vi "List-ALL-subfolders-and-files-1D.vi"(7 "pattern":string="*", 8 "error in":errorcluster, 11 "Top level folder":path=path "/user/pma") -> (0 "error IO":errorcluster, 2 "Folders accessed":path[](array[path]), 3 "files found":path[](array[path]))   [LabVIEW 2014]
panel:
  out "Found":i32
  # "This VI lists all files in all subfolders\nstarting from top level folder\nand down. Can be filtered by pattern"
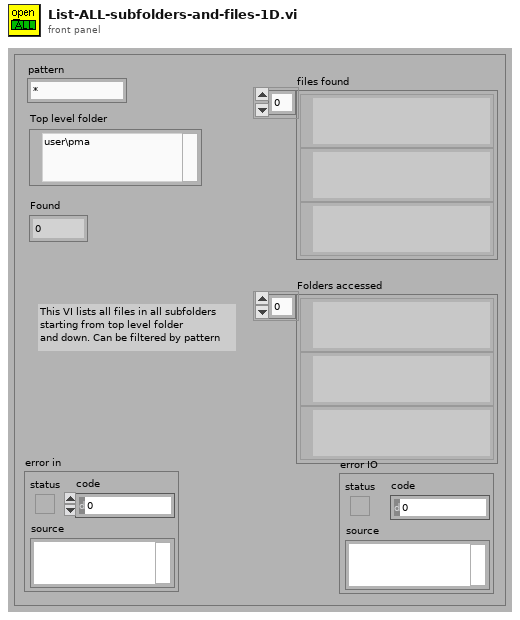
[diagram p1: front panel]
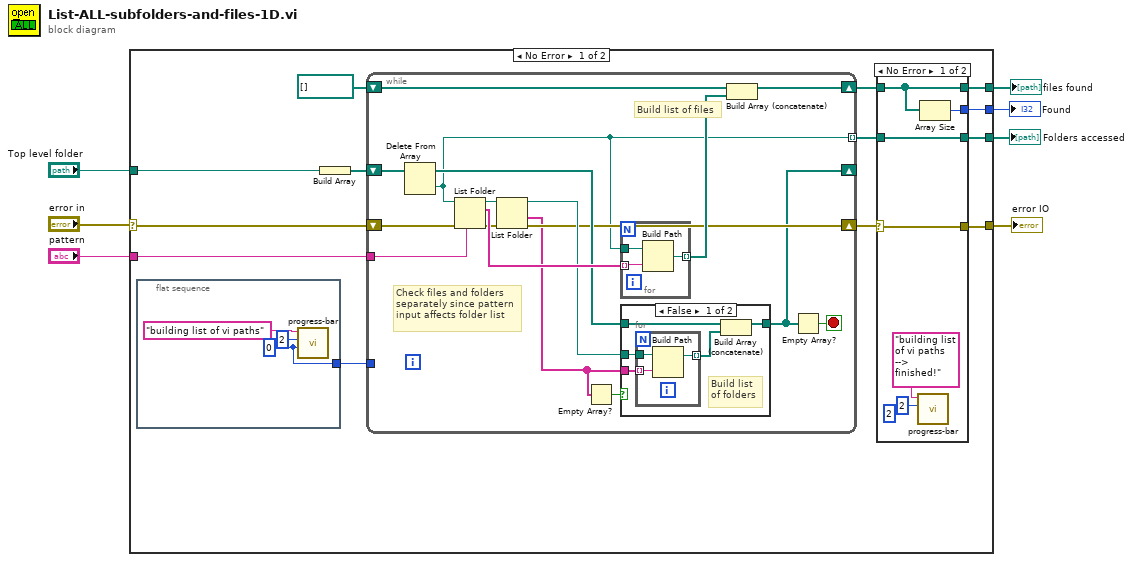
[diagram p0: block diagram]
diagram:
  n1 = case shown="No Error" "error in" {
    selector: "error in" -> [w17 w60]
    tunnel: "Top level folder" -> [w20 _]
    tunnel: [w11 _] -> w6
    tunnel: [w10 _] -> w5
    tunnel: [w9 w60] -> w2
    tunnel: [w13 _] -> w4
    tunnel: "pattern" -> [w16 _]
    frame No Error {
      n2 = flat-sequence {
        tunnel: [w21] -> w8
        frame #0 {
          w21 = u32 0 ("i++")
          n3 = call "progress-bar.vi"("i++"=w21, "max"=2, "state"="building list of vi paths") -> ()  [unwired: 9 out]
        }
      }
      n4 = Build Array(w20) -> (w19:path[])
      n5 = while {
        shift-left: path[] [] ("Array Constant") -> [w44]
        shift-right: [w47] -> w12
        shift-left: w19 -> [w46]
        shift-right: [w35] -> _
        shift-right: [w40] -> w15
        shift-left: w17 -> [w39]
        tunnel: [w33] -> w14 mode=indexing
        tunnel: w16 -> [w38]
        tunnel: w8 -> [_]
        stop <- w34 stop-if-true
        # "Check files and folders\nseparately since pattern\ninput affects folder list"
        # "Build list of files"
        n6 = Delete From Array(array=w46) -> (deleted portion=w33:path, array with subset deleted=w42:path[])  [unwired: 2 in]
        n7 = List Folder(path=w33, pattern=w38, error in=w39) -> (path out=w31:path, filenames=w45:string[], error out=w32:errorcluster)  [unwired: 2 out]
        n8 = List Folder(path=w31, error in=w32) -> (path out=w41:path, folder names=w37:string[], error out=w40:errorcluster)  [unwired: 3 out]
        n9 = Empty Array?(array=w37) -> (empty?=w36:bool)
        n10 = for {
          tunnel: w45 -> [w58] mode=indexing
          tunnel: w33 -> [w59]
          tunnel: [w57] -> w43 mode=indexing
          n11 = Build Path(base path=w59, name or relative path=w58) -> (appended path=w57:path)
        }
        n12 = case shown="False" w36 {
          tunnel: w42 -> [w50 w56]
          tunnel: [w51 w56] -> w35
          tunnel: w41 -> [w52 _]
          tunnel: w37 -> [w48 _]
          frame False {
            # "Build list\nof folders"
            n13 = for {
              tunnel: w52 -> [w55]
              tunnel: [w54] -> w49 mode=indexing
              tunnel: w48 -> [w53] mode=indexing
              n14 = Build Path(base path=w55, name or relative path=w53) -> (appended path=w54:path)
            }
            n15 = Build Array (concatenate)(w50, w49) -> (w51:path[])
          }
          frame True {
          }
        }
        n16 = Build Array (concatenate)(w44, w43) -> (w47:path[])
        n17 = Empty Array?(array=w35) -> (empty?=w34:bool)
      }
      n18 = case shown="No Error" w15 {
        selector: w15 -> [w26 w30]
        tunnel: w14 -> [w29 _]
        tunnel: [w29 _] -> w13
        tunnel: w12 -> [w28 _]
        tunnel: [w28 _] -> w11
        tunnel: [w27 _] -> w10
        tunnel: [w26 w30] -> w9
        frame No Error {
          (unwired) u32 2 ("i++")
          n19 = call "progress-bar.vi"("max"=2, "state"="building list of vi paths --> finished!") -> ()  [unwired: 1 in, 9 out]
          n20 = Array Size(array=w28) -> (size(s)=w27:i32)
        }
        frame Error {
          # "Output empty\narrays if an\nerror occurred\nduring the list"
        }
      }
    }
    frame Error {
    }
  }
  "files found" <- w6
  "Found" <- w5
  "Folders accessed" <- w4
  "error IO" <- w2
